vi "SetMessageBrokerError.vi"(8 "error in (no error)":errorcluster, 10 "Message Broker Errors":T1, 11 "Message Broker in":refnum<class "Message Broker.lvclass">) -> (0 "error out":errorcluster, 3 "Message Broker out":refnum<class "Message Broker.lvclass">)   [LabVIEW 2016, in "Stream Mediator.lvlib" / "Message Broker.lvclass"]
doc: "--\nCopyright © 2017 Composed SystemsI All rights reserved.\n\nAuthor: Jon McBee <jon.mcbee@composed.io>\n\nThis library is provided \"AS IS\" ,WITHOUT WARRANTIES OR\nCONDITIONS OF ANY KIND, either express or implied.\n\nComposed Systems -- composed.io\n\nStream 0.0.1.1\nJon McBee - Composed Systems\nCopyright (c) 2017, Composed Systems"
uses:
  <userlib>/Composed Systems/Stream/Mediator/Classes/Message Broker/Message Broker.lvclass
  <userlib>/Composed Systems/Stream/Mediator/Classes/Message Broker/MessageBrokerErrors.ctl
  <vilib>/Utility/error.llb/Error Cluster From Error Code.vi
  <vilib>/ErrorRing/Error Ring.xnode
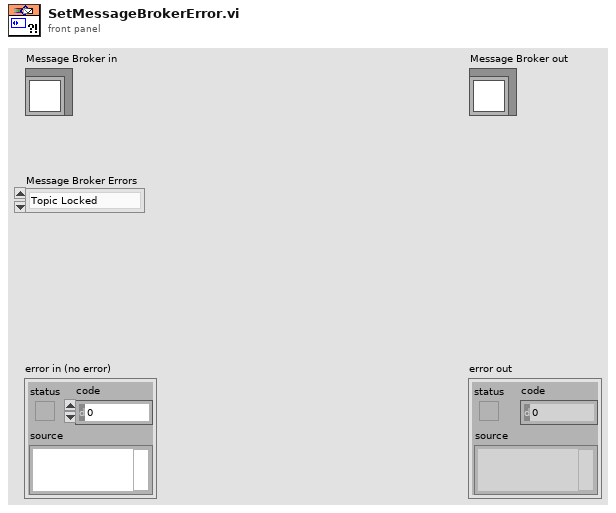
[diagram p1: front panel]
types:
  T1 = typedef "Stream Mediator.lvlib/Message Broker.lvclass/MessageBrokerErrors.ctl" = enum16{"Topic Locked"}
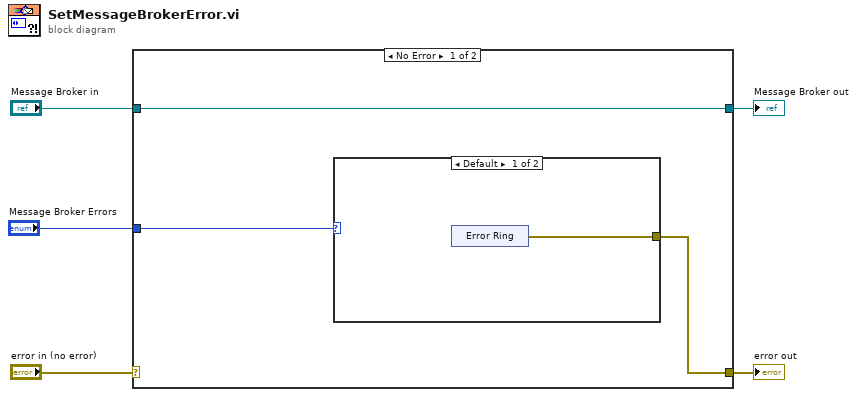
[diagram p0: block diagram]
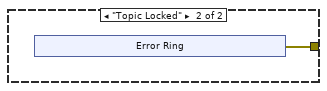
[diagram p2: hidden frame]
diagram:
  n1 = case shown="No Error" "error in (no error)" {
    selector: "error in (no error)" -> [_ w18]
    tunnel: [w6 w18] -> w4
    tunnel: [w8 w17] -> w2
    tunnel: "Message Broker in" -> [w8 w17]
    tunnel: "Message Broker Errors" -> [w7 _]
    frame No Error {
      n2 = case shown="Default" w7 {
        tunnel: [w9 w11] -> w6
        frame Default {
          n3 = xnode "Error Ring"() -> ("error out"=w9:errorcluster)
        }
        frame "Topic Locked" {
          n4 = xnode "Error Ring"() -> ("error out"=w11:errorcluster)
        }
      }
    }
    frame Error {
    }
  }
  "error out" <- w4
  "Message Broker out" <- w2
